vi "装饰模式DEMO.vi"() -> ()   [LabVIEW 2013]
uses:
  Motor_class/Motor.lvclass
  Direction_class/Direction.lvclass
  Speed_class/Speed.lvclass
panel:
  out "Output":string
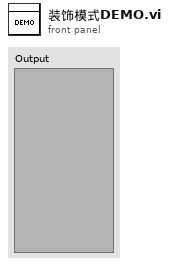
[diagram p1: front panel]
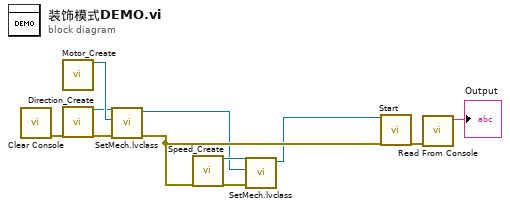
[diagram p0: block diagram]
diagram:
  n1 = call "Clear Console.vi"() -> ("error out"=w8:errorcluster)  [unwired: 11 in]
  n2 = call "Motor_Create.vi"() -> ("reference out"=w7:refnum<class "Motor.lvclass">)  [unwired: 18 in, 1 out]
  n3 = call "Direction_Create.vi"("error in (no error)"=w8) -> ("reference out"=w6:refnum<class "Direction.lvclass">, "error out"=w11:errorcluster)  [unwired: 17 in]
  n4 = call-dynamic "SetMech.lvclass.vi"("error in (no error)"=w11, "Mech.lvclass"=w7, "reference in"=w6) -> ("error out"=w5:errorcluster, "reference out"=w2:refnum<class "Direction.lvclass">)  [unwired: 7 in]
  n5 = call "Speed_Create.vi"("error in (no error)"=w5) -> ("reference out"=w3:refnum<class "Speed.lvclass">, "error out"=w4:errorcluster)  [unwired: 17 in]
  n6 = call-dynamic "SetMech.lvclass.vi"("error in (no error)"=w4, "Mech.lvclass"=w2, "reference in"=w3) -> ("reference out"=w1:refnum<class "Speed.lvclass">)  [unwired: 7 in, 1 out]
  n7 = call-dynamic "Start.vi"("reference in"=w1, "error in (no error)"=w5) -> ("error out"=w10:errorcluster)  [unwired: 16 in, 1 out]
  n8 = call "Read From Console.vi"("error in (no error)"=w10) -> ("Output"=→"Output":string)  [unwired: 9 in, 1 out]
